vi "ExSubCreateImageDisplay.vi"(0 "Camera Handle":u32, 1 "File and Display Name":string, 2 "error in (no error)":errorcluster) -> (3 "Camera Handle":u32, 4 "Display Handle":u32, 5 "Image Handle":u32, 6 "error out":errorcluster)   [LabVIEW 2010]
panel:
  # "ExSubCreateImageDisplay:\nThis is a SubVI that creates a file, display and image \nobjects and returns the handles bundled in a cluster \nthat includes and camera handle"
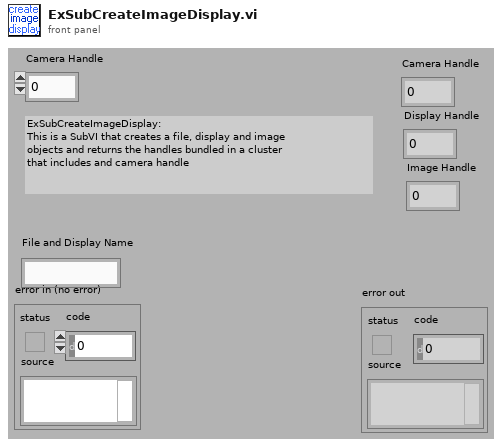
[diagram p1: front panel]
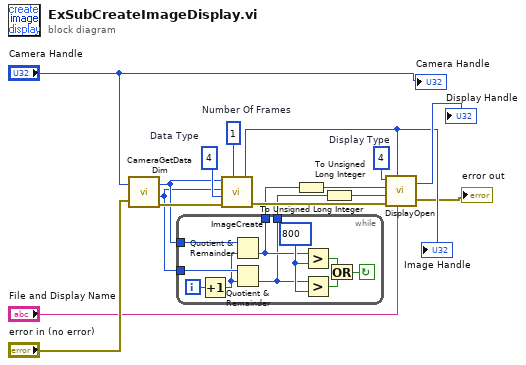
[diagram p0: block diagram]
diagram:
  w11 = u32 1  # Number Of Frames
  w12 = u32 4  # Display Type
  w13 = u32 4  # Data Type
  n1 = call <userlib>:"CameraGetDataDim.vi"("Camera Handle"="Camera Handle", "error in"="error in (no error)") -> ("Xdim"=w10:u32, "Ydim"=w9:u32, "error out"=w17:errorcluster)  [unwired: 1 out]
  n2 = while {
    tunnel: w10 -> [w26]
    tunnel: w9 -> [w25]
    tunnel: [w20] -> w8
    tunnel: [w19] -> w7
    i -> [w24]
    stop <- w21 continue-if-true
    w27 = 800
    n3 = Increment(x=w24) -> (x+1=w18:i32)
    n4 = Quotient & Remainder(x=w26, y=w18) -> (floor(x/y)=w20:u32)  [unwired: 1 out]
    n5 = Quotient & Remainder(x=w25, y=w18) -> (floor(x/y)=w19:u32)  [unwired: 1 out]
    n6 = Greater?(x=w20, y=w27) -> (0:w23:bool)
    n7 = Greater?(x=w19, y=w27) -> (0:w22:bool)
    n8 = Or(x=w23, y=w22) -> (x .or. y?=w21:bool)
  }
  n9 = call <userlib>:"ImageCreate.vi"("X dimension"=w10, "Y dimension"=w9, "Data Type"=w13, "error in"=w17, "Number Of Frames"=w11) -> ("Image Handle"=w2:u32, "error out"=w16:errorcluster)
  "Image Handle" <- w2
  n10 = To Unsigned Long Integer(number=w8) -> (unsigned 32bit integer=w6:u32)
  n11 = To Unsigned Long Integer(number=w7) -> (unsigned 32bit integer=w5:u32)
  n12 = call <userlib>:"DisplayOpen.vi"("Display Title"="File and Display Name", "Image Handle"=w2, "error in"=w16, "Display Height"=w5, "Display Width"=w6, "Display Type"=w12) -> ("error out"=→"error out":errorcluster, "Display Handle"=→"Display Handle":u32)
  "Camera Handle" <- "Camera Handle"
